vi "Library Initialize and Exit.vi"(7 "action":enum16{"LibInit", "LibExit"}(ring), 8 "error in":errorcluster) -> (0 "error out":errorcluster, 1 "modules found":i32, 3 "instance count":i32)   [LabVIEW 2020, in "AIM ARINC 429 Hardware API.lvlib"]
uses:
  AIM ARINC 429 Hardware API.lvlib
  <instrlib>/_AIM 429/AIM429LV.lvlib
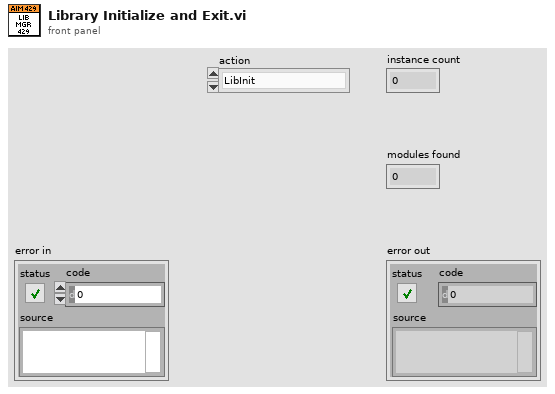
[diagram p1: front panel]
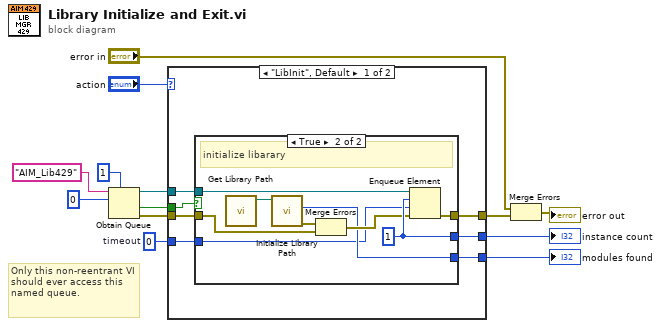
[diagram p0: block diagram]
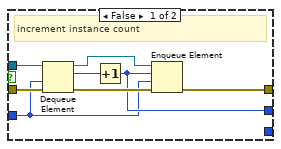
[diagram p2: hidden frame]
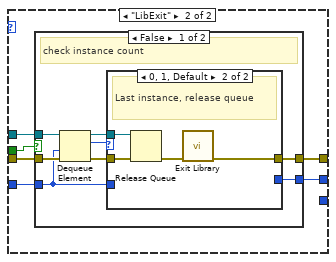
[diagram p3: hidden frame]
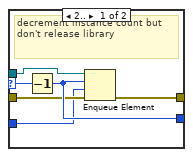
[diagram p4: hidden frame]
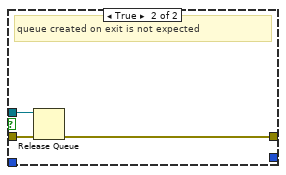
[diagram p5: hidden frame]
diagram:
  w1 = 0  # timeout
  # "Only this non-reentrant VI should ever access this named queue."
  n1 = Obtain Queue(max queue size (-1, unlimited)=1, name (unnamed)="AIM_Lib429", element data type=0) -> (queue out=w4:refnum<queue>, created new?=w3:bool, error out=w2:errorcluster)  [unwired: 2 in]
  n2 = case shown="\"LibInit\", Default" "action" {
    tunnel: [w20 w43] -> w11
    tunnel: [w19 w42] -> w13
    tunnel: [w18 _] -> w12
    tunnel: w4 -> [w17 w41]
    tunnel: w3 -> [w16 w40]
    tunnel: w2 -> [w15 w39]
    tunnel: w1 -> [w14 w38]
    frame "LibInit", Default {
      n3 = case shown="True" w16 {
        tunnel: w15 -> [w27 w33]
        tunnel: [w24 w37] -> w20
        tunnel: [w23 w35] -> w19
        tunnel: w17 -> [w28 w36]
        tunnel: [_ w32] -> w18
        tunnel: w14 -> [w21 w30]
        frame False {
          # "increment instance count"
          n4 = Dequeue Element(queue=w28, timeout in ms (-1)=w21, error in (no error)=w27) -> (queue out=w26:refnum<queue>, element=w22:i32, error out=w25:errorcluster)  [unwired: 1 out]
          n5 = Increment(x=w22) -> (x+1=w23:i32)
          n6 = Enqueue Element(queue=w26, element=w23, timeout in ms (-1)=w21, error in (no error)=w25) -> (error out=w24:errorcluster)  [unwired: 2 out]
        }
        frame True {
          w35 = 1 ("modules found")
          # "initialize libarary"
          n7 = call <instrlib>:"Get Library Path.vi"() -> ("GlobalDLLPath"=w29:path)  [unwired: 11 in]
          n8 = call "Initialize Library Path.vi"("library path"=w29) -> ("error out"=w31:errorcluster, "modules found"=w32:i32)  [unwired: 9 in]
          n9 = Merge Errors(w31, w33) -> (w34:errorcluster)
          n10 = Enqueue Element(queue=w36, element=w35, timeout in ms (-1)=w30, error in (no error)=w34) -> (error out=w37:errorcluster)  [unwired: 2 out]
        }
      }
    }
    frame "LibExit" {
      n11 = case shown="False" w40 {
        tunnel: [w51 w62] -> w43
        tunnel: [w50 _] -> w42
        tunnel: w41 -> [w49 w64]
        tunnel: w39 -> [w48 w63]
        tunnel: w38 -> [w44 _]
        frame False {
          # "check instance count"
          n12 = Dequeue Element(queue=w49, timeout in ms (-1)=w44, error in (no error)=w48) -> (queue out=w46:refnum<queue>, element=w47:i32, error out=w45:errorcluster)  [unwired: 1 out]
          n13 = case shown="0, 1, Default" w47 {
            selector: w47 -> [w55 _]
            tunnel: [w56 w58] -> w51
            tunnel: [w57 _] -> w50
            tunnel: w46 -> [w54 w61]
            tunnel: w45 -> [w53 w60]
            tunnel: w44 -> [w52 _]
            frame 2.. {
              # "decrement instance count but don't release library"
              n14 = Decrement(x=w55) -> (x-1=w57:i32)
              n15 = Enqueue Element(queue=w54, element=w57, timeout in ms (-1)=w52, error in (no error)=w53) -> (error out=w56:errorcluster)  [unwired: 2 out]
            }
            frame 0, 1, Default {
              # "Last instance, release queue"
              n16 = Release Queue(queue=w61, error in (no error)=w60) -> (error out=w59:errorcluster)  [unwired: 1 in, 2 out]
              n17 = call "Exit Library.vi"("error in"=w59) -> ("error out"=w58:errorcluster)  [unwired: 9 in, 1 out]
            }
          }
        }
        frame True {
          # "queue created on exit is not expected"
          n18 = Release Queue(queue=w64, error in (no error)=w63) -> (error out=w62:errorcluster)  [unwired: 1 in, 2 out]
        }
      }
    }
  }
  "instance count" <- w13
  "modules found" <- w12
  n19 = Merge Errors("error in", w11) -> (→"error out":errorcluster)
